vi "Unloading_Empty_Bin_Check.vi"(7 "Cluster DATA IN":T1, 8 "error in (no error)":errorcluster) -> (0 "error out":errorcluster, 2 "EMPTY FOUND ?":bool, 5 "Cluster DATA OUT":T1)   [LabVIEW 2017]
uses:
  Controls/Unload_Cyc_Data.ctl
  <vilib>/Utility/file.llb/Read Delimited Spreadsheet (string).vi
panel:
  # "UNLOAD"
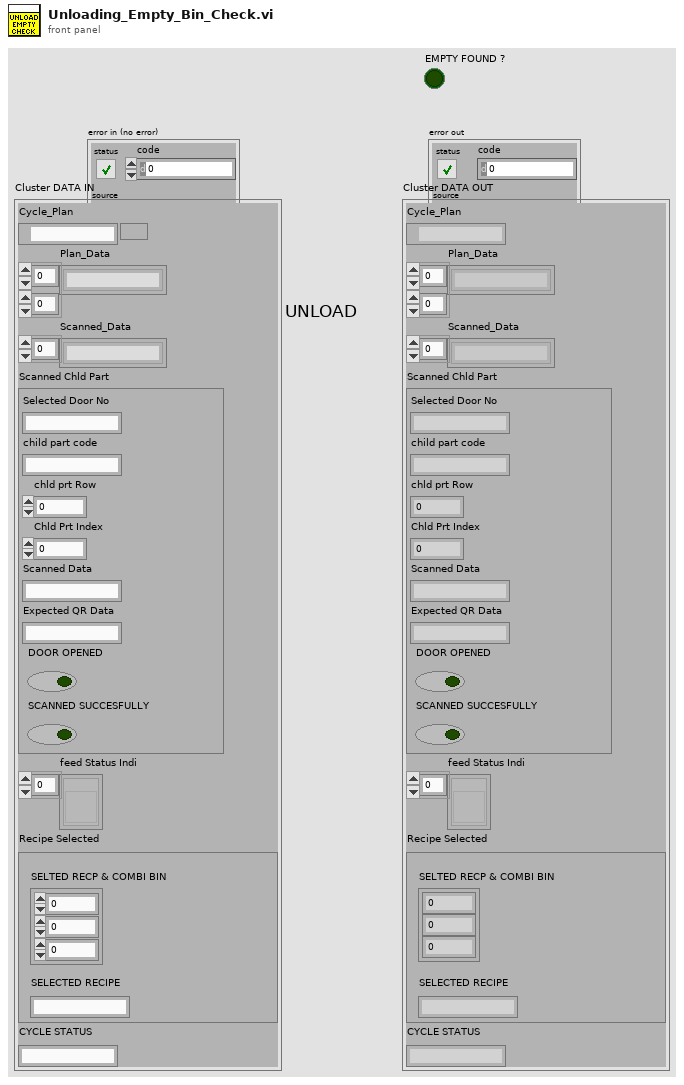
[diagram p1: front panel]
types:
  T1 = typedef "Unload_Cyc_Data.ctl" = cluster{"Cycle_Plan":path, "Plan_Data":string[][], "Scanned_Data":string[], "Scanned Chld Part":cluster{"Selected Door No":string, "child part code":string, "chld prt Row":i32, "Chld Prt Index":i32, "Scanned Data":string, "Expected QR Data":string, "DOOR OPENED":bool, "SCANNED SUCCESFULLY":bool}, "feed Status Indi":refnum<vi>[], "Recipe Selected":cluster{"SELTED RECP & COMBI BIN":cluster{"RECIPE INDEX":i32, "COMBI BIN":i32, "Section row no.":i32}, "SELECTED RECIPE":string}, "CYCLE STATUS":string}
  T2 = cluster{"RECIPE INDEX":i32, "COMBI BIN":i32, "Section row no.":i32}
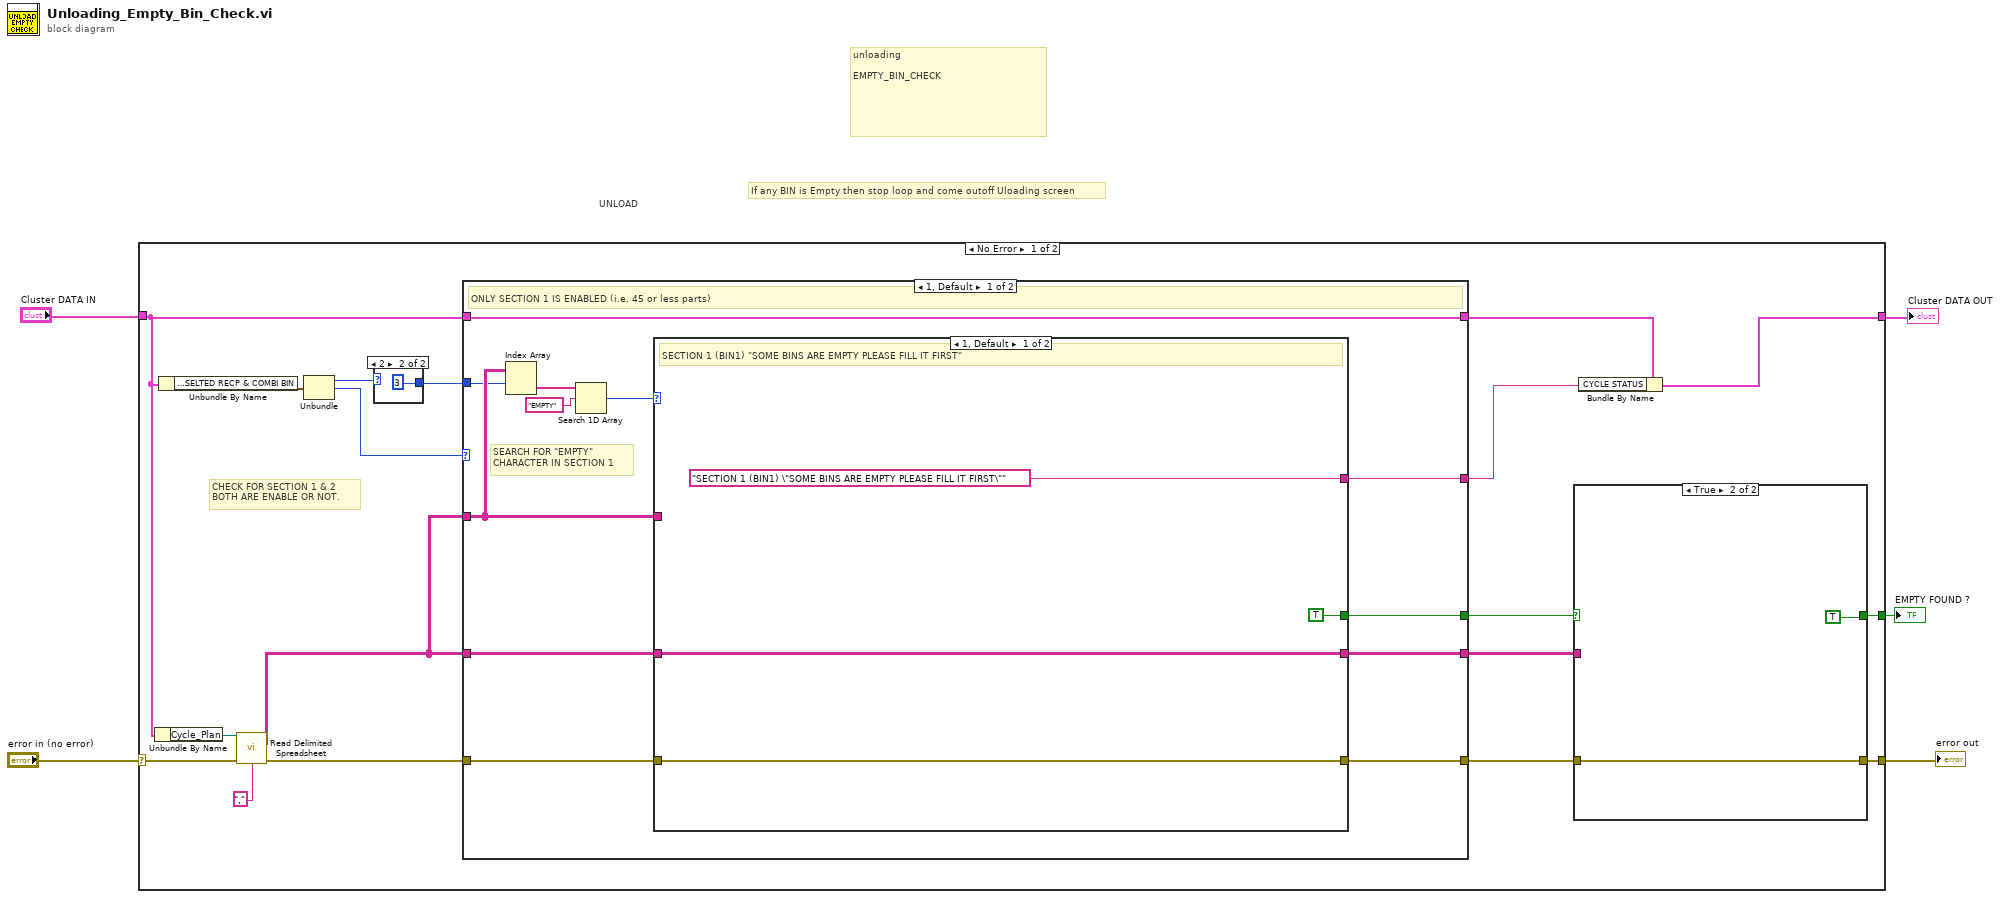
[diagram p0: block diagram]
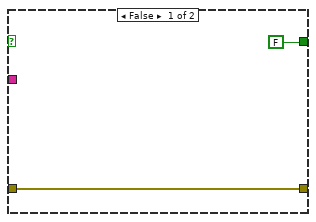
[diagram p2: hidden frame]
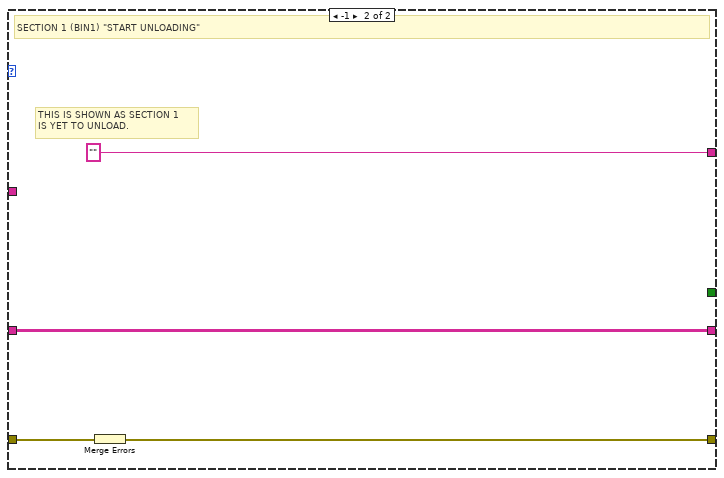
[diagram p3: hidden frame]
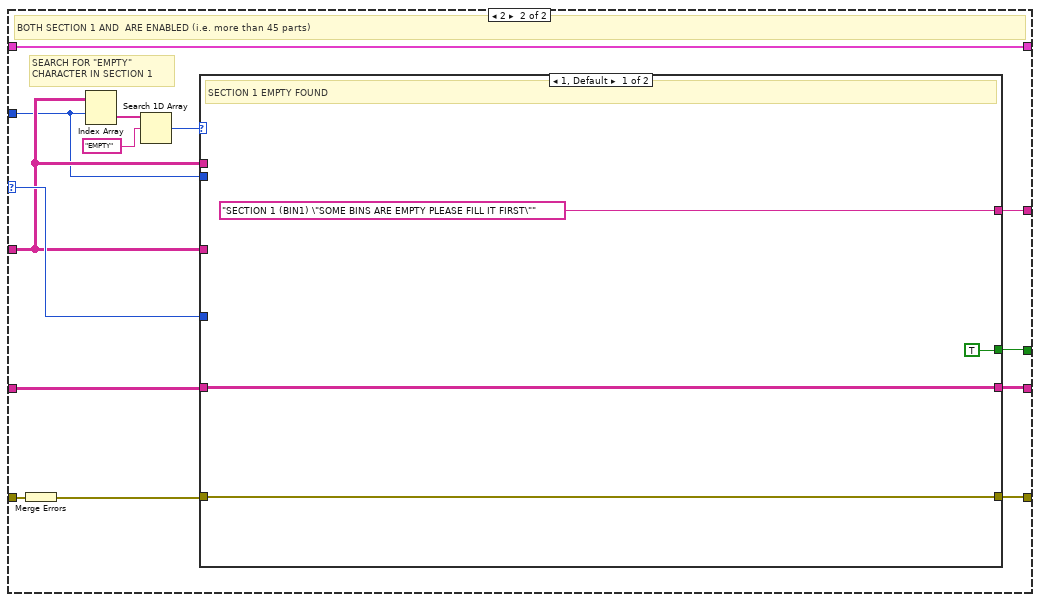
[diagram p4: hidden frame]
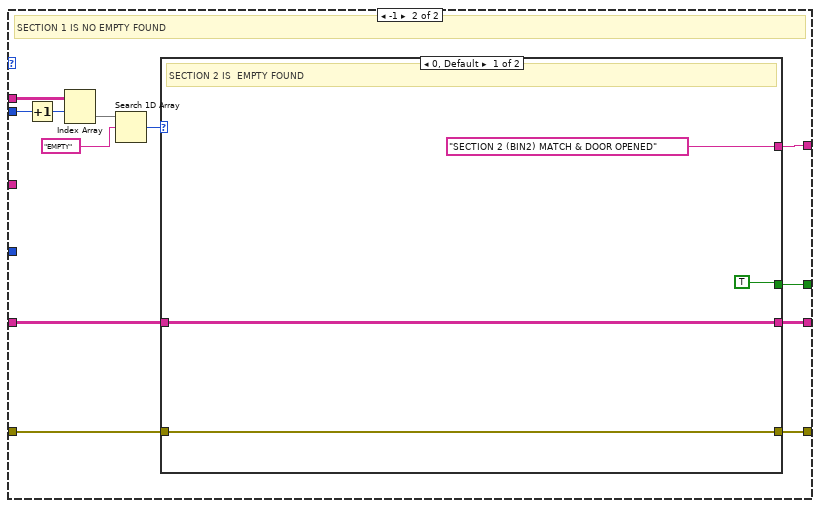
[diagram p5: hidden frame]
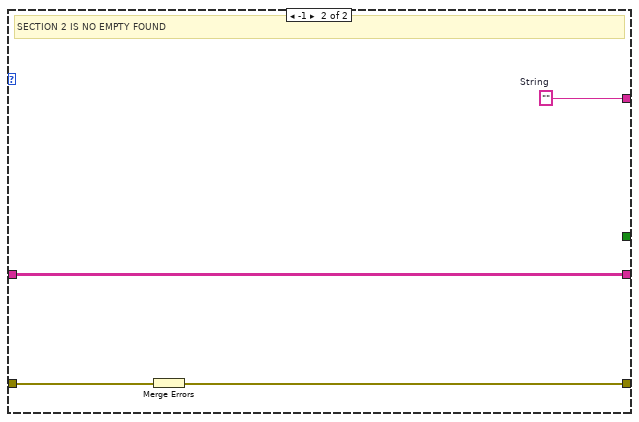
[diagram p6: hidden frame]
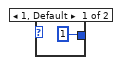
[diagram p7: hidden frame]
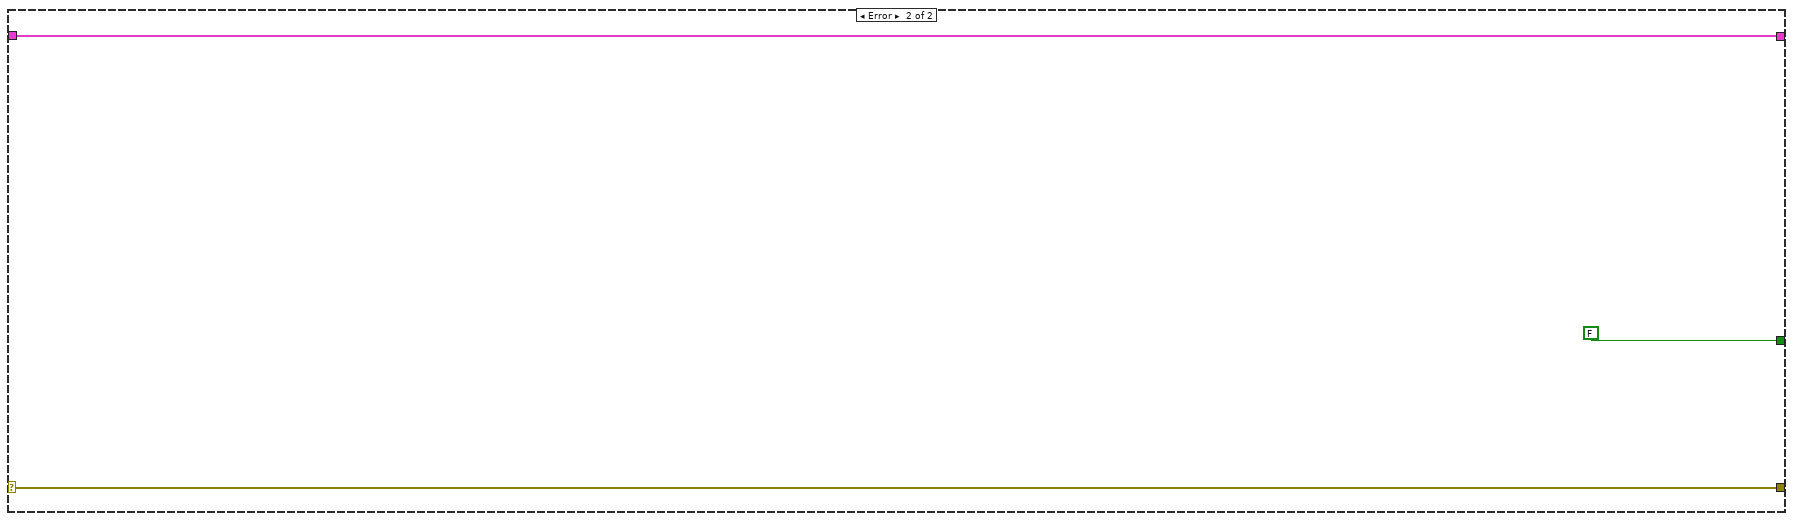
[diagram p8: hidden frame]
diagram:
  # "UNLOAD"
  # "If any BIN is Empty then stop loop and come outoff Uloading screen"
  # "unloading\n\nEMPTY_BIN_CHECK"
  n1 = case shown="No Error" "error in (no error)" {
    selector: "error in (no error)" -> [w20 w90]
    tunnel: [w12 w90] -> w4
    tunnel: [w7 w89] -> w2
    tunnel: "Cluster DATA IN" -> [w16 w89]
    tunnel: [w9 FALSE] -> w1
    frame No Error {
      # "CHECK FOR SECTION 1 & 2\nBOTH ARE ENABLE OR NOT."
      n2 = Unbundle By Name(w16) -> ("Cycle_Plan"=w21:path)
      n3 = Unbundle By Name(w16) -> ("Recipe Selected.SELTED RECP & COMBI BIN"=w18:T2)
      n4 = call-poly <vilib>:"Read Delimited Spreadsheet.vi"("file path (dialog if empty)"=w21, "error in (no error)"=w20, "delimiter (\\t)"=",") -> ("all rows"=w14:string[][], "error out"=w19:errorcluster)  [unwired: 7 in, 4 out]
      n5 = Unbundle(w18) -> ("RECIPE INDEX"=w17:i32, "COMBI BIN"=w13:i32)  [unwired: 1 out]
      n6 = case shown="2" w17 {
        tunnel: [1 3] -> w15
        frame 1, Default {
        }
        frame 2 {
        }
      }
      n7 = case shown="1, Default" w13 {
        selector: w13 -> [_ w51]
        tunnel: [w38 w57] -> w23
        tunnel: w19 -> [w39 w61]
        tunnel: [w37 w60] -> w8
        tunnel: w16 -> [w37 w60]
        tunnel: w14 -> [w34 w49]
        tunnel: w15 -> [w31 w48]
        tunnel: w14 -> [w36 w59]
        tunnel: [w35 w56] -> w10
        tunnel: [w33 w55] -> w11
        tunnel: [w32 w54] -> w6
        frame 1, Default {
          # "SEARCH FOR \"EMPTY\"\nCHARACTER IN SECTION 1"
          # "ONLY SECTION 1 IS ENABLED (i.e. 45 or less parts)"
          n8 = Index Array(array=w34, index (row)=w31) -> (element=w30:string[])  [unwired: 1 in]
          n9 = Search 1D Array(1D array=w30, element="EMPTY") -> (index of element=w28:i32)  [unwired: 1 in]
          n10 = case shown="1, Default" w28 {
            tunnel: w39 -> [w43 w47]
            tunnel: [w43 w46] -> w38
            tunnel: w36 -> [w42 w45]
            tunnel: [w42 w45] -> w35
            tunnel: w34 -> [_ _]
            tunnel: [TRUE _] -> w33
            tunnel: ["SECTION 1 (BIN1) \"SOME BINS ARE EMPTY PLEASE FILL IT FIRST\"" ""] -> w32
            frame 1, Default {
              # "SECTION 1 (BIN1) \"SOME BINS ARE EMPTY PLEASE FILL IT FIRST\""
            }
            frame -1 {
              # "THIS IS SHOWN AS SECTION 1\nIS YET TO UNLOAD."
              # "SECTION 1 (BIN1) \"START UNLOADING\""
              n11 = Merge Errors(w47) -> (w46:errorcluster)
            }
          }
        }
        frame 2 {
          # "SEARCH FOR \"EMPTY\"\nCHARACTER IN SECTION 1"
          # "BOTH SECTION 1 AND  ARE ENABLED (i.e. more than 45 parts)"
          n12 = Merge Errors(w61) -> (w58:errorcluster)
          n13 = Index Array(array=w49, index (row)=w48) -> (element=w53:string[])  [unwired: 1 in]
          n14 = Search 1D Array(1D array=w53, element="EMPTY") -> (index of element=w50:i32)  [unwired: 1 in]
          n15 = case shown="1, Default" w50 {
            tunnel: [w65 w76] -> w57
            tunnel: w58 -> [w65 w77]
            tunnel: [w64 w75] -> w56
            tunnel: w59 -> [w64 w74]
            tunnel: w49 -> [_ _]
            tunnel: w51 -> [_ _]
            tunnel: [TRUE w73] -> w55
            tunnel: ["SECTION 1 (BIN1) \"SOME BINS ARE EMPTY PLEASE FILL IT FIRST\"" w67] -> w54
            tunnel: w49 -> [_ w72]
            tunnel: w48 -> [_ w71]
            frame 1, Default {
              # "SECTION 1 EMPTY FOUND"
            }
            frame -1 {
              # "SECTION 1 IS NO EMPTY FOUND"
              n16 = Increment(x=w71) -> (x+1=w70:i32)
              n17 = Index Array(array=w72, index (row)=w70) -> (element=w69:string[])  [unwired: 1 in]
              n18 = Search 1D Array(1D array=w69, element="EMPTY") -> (index of element=w66:i32)  [unwired: 1 in]
              n19 = case shown="0, Default" w66 {
                tunnel: w77 -> [w81 w85]
                tunnel: [w81 w84] -> w76
                tunnel: [w80 w83] -> w75
                tunnel: w74 -> [w80 w83]
                tunnel: [TRUE _] -> w73
                tunnel: ["SECTION 2 (BIN2) MATCH & DOOR OPENED" w82] -> w67
                frame 0, Default {
                  # "SECTION 2 IS  EMPTY FOUND"
                }
                frame -1 {
                  w82 = ""  # String
                  # "SECTION 2 IS NO EMPTY FOUND"
                  n20 = Merge Errors(w85) -> (w84:errorcluster)
                }
              }
            }
          }
        }
      }
      n21 = case shown="True" w11 {
        tunnel: w23 -> [w25 w27]
        tunnel: [w25 w27] -> w12
        tunnel: w10 -> [_ _]
        tunnel: [FALSE TRUE] -> w9
        frame False {
        }
        frame True {
        }
      }
      n22 = Bundle By Name(cluster=w8, "CYCLE STATUS"=w6) -> (w7:T1)
    }
    frame Error {
    }
  }
  "error out" <- w4
  "Cluster DATA OUT" <- w2
  "EMPTY FOUND ?" <- w1
